vi "SetCollectorDataStructure.vi"(8 "error in (no error)":errorcluster, 11 "DataCollector in":refnum<class "DataCollector.lvclass">) -> (0 "error out":errorcluster, 3 "DataCollector out":refnum<class "DataCollector.lvclass">)   [LabVIEW 2017, in "DataCollector.lvclass"]
uses:
  DataCollector.lvclass
  DataCollector.lvclass/DataCollector.ctl
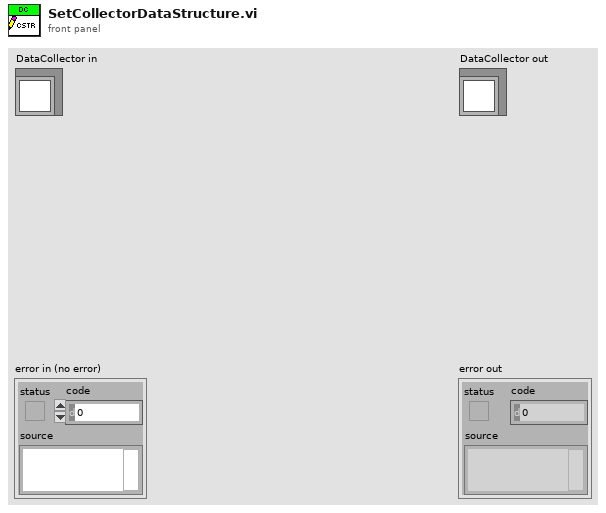
[diagram p1: front panel]
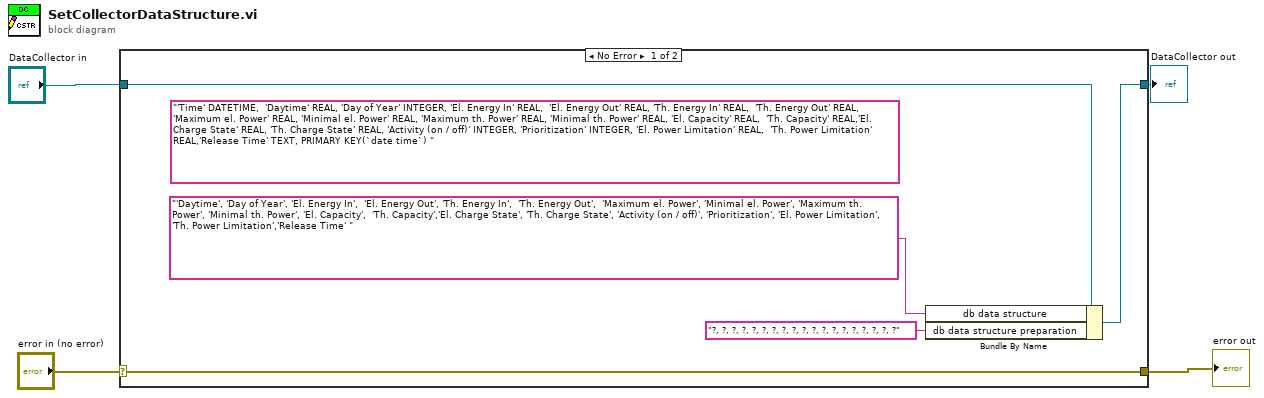
[diagram p0: block diagram]
diagram:
  n1 = case shown="No Error" "error in (no error)" {
    selector: "error in (no error)" -> [w9 w10]
    tunnel: [w9 w10] -> w3
    tunnel: [w7 w11] -> w1
    tunnel: "DataCollector in" -> [w8 w11]
    frame No Error {
      (unwired) "'Time' DATETIME,  'Daytime' REAL, 'Day of Year' INTEGER, 'El. Energy In' REAL,  'El. Energy Out' REAL, 'Th. Energy In' REAL,  'Th. Energy Out' REAL,  'Maximum el. Power' REAL, 'Minimal el. Power' REAL, 'Maximum th. Power' REAL, 'Minimal th. Power' REAL, 'El. Capacity' REAL,  'Th. Capacity' REAL,'El. Charge State' REAL, 'Th. Charge State' REAL, 'Activity (on / off)' INTEGER, 'Prioritization' INTEGER, 'El. Power Limitation' REAL,  'Th. Power Limitation' REAL,'Release Time' TEXT, PRIMARY KEY(`date time`) " ("string")
      n2 = Bundle By Name(cluster=w8, "db data structure"="'Daytime', 'Day of Year', 'El. Energy In',  'El. Energy Out', 'Th. Energy In',  'Th. Energy Out',  'Maximum el. Power', 'Minimal el. Power', 'Maximum th. Power', 'Minimal th. Power', 'El. Capacity',  'Th. Capacity','El. Charge State', 'Th. Charge State', 'Activity (on / off)', 'Prioritization', 'El. Power Limitation',  'Th. Power Limitation','Release Time' " ("string"), "db data structure preparation"="?, ?, ?, ?, ?, ?, ?, ?, ?, ?, ?, ?, ?, ?, ?, ?, ?, ?, ?") -> (w7:refnum<class "DataCollector.lvclass">)
    }
    frame Error {
    }
  }
  "error out" <- w3
  "DataCollector out" <- w1
